vi "Actor Core.vi"(8 "error in":errorcluster, 11 "Create Test Channel View in":refnum<class "Edit Test Channel View.lvclass">) -> (0 "error out":errorcluster, 3 "Actor out":refnum<class "Actor.lvclass">)   [LabVIEW 2013, in "Edit Test Channel View.lvlib" / "Edit Test Channel View.lvclass"]
doc: "(<B>Filename</B>: Actor Framework.lvlib:Actor.lvclass:Actor Core.vi)\n\nReceives messages to the actor, reacts to them, and initiates any error handling that may shut the actor down.\n\nDescendant classes may override this VI to append parallel tasks for the actor to complete while it handles messages. Overrides use the Call Parent Method node."
uses:
  Edit Test Channel View.lvclass
  <vilib>/ActorFramework/Actor/Actor.lvclass
  <vilib>/ActorFramework/Actor/Actor.lvclass/Actor.ctl
  <vilib>/ActorFrameworkMVC/View Actor/View Actor.lvclass
  <vilib>/ActorFramework/Message Enqueuer/Message Enqueuer.lvclass/Message Enqueuer.ctl
  Edit Test Channel View.lvclass/Edit Test Channel View.ctl
  Models/Edit Test Channel Model Messages/Set Item Configurations Msg/Set Item Configurations Msg.lvclass/Set Item Configurations Msg.ctl
  <vilib>/Utility/miscctls.llb/LVPositionTypeDef.ctl
  <vilib>/ActorFrameworkMVC/UI Controller Messages/Move Subpanel Msg/Move Subpanel Msg.lvclass/Move Subpanel Msg.ctl
  <vilib>/ActorFrameworkMVC/UI Controller Messages/Insert Subpanel Msg/Insert Subpanel Msg.lvclass/Insert Subpanel Msg.ctl
  <vilib>/ActorFramework/Message Enqueuer/Init from Existing Queue.vi
  <vilib>/ActorFramework/Message Enqueuer/Enqueue.vi
  <vilib>/ActorFramework/Message Priority Queue/Priority Enqueue.vi
  <vilib>/ActorFramework/Message Enqueuer/Message Enqueuer.lvclass
  Models/Edit Test Channel Model Messages/Set Item Configurations Msg/Set Item Configurations Msg.lvclass
  Models/Edit Test Channel Model Messages/Load Test Channel Msg/Load Test Channel Msg.lvclass
  <vilib>/ActorFrameworkMVC/UI Controller Messages/Move Subpanel Msg/Move Subpanel Msg.lvclass
  <vilib>/ActorFrameworkMVC/UI Controller Messages/Insert Subpanel Msg/Insert Subpanel Msg.lvclass
  Models/Edit Test Channel Model Messages/Save Test Channel Msg/Save Test Channel Msg.lvclass
  Models/Test Channel Model Messages/Preview Test Channel Msg/Preview Test Channel Msg.lvclass
  Models/Test Channel Model Messages/Update Tiles Info Msg/Update Tiles Info Msg.lvclass
  Models/Test Channel Model Messages/Update Previous Button Visibility Msg/Update Previous Button Visibility Msg.lvclass
  Models/Test Channel Model Messages/Update Next Button Visibility Msg/Update Next Button Visibility Msg.lvclass
  Common/File IO/File IO.lvlib
  <vilib>/ActorFrameworkMVC/View Actor Messages/Get Model Enqueuer Msg/Get Model Enqueuer Msg.lvclass
  <vilib>/ActorFrameworkMVC/UI Controller Messages/Get Model Actor Enqueuer Msg/Get Model Actor Enqueuer Msg.lvclass
panel:
  in  "Cancel":bool
  in  "Save":bool
  out "Tab Control":enum32{"Basic Info"}(tab)
  in  "Channel Description":string caption="测试通道描述："
  in  "Channel Name":string caption="测试通道名称："
  in  "Channel ID":u16(ring) caption="测试通道ID：" items=["通道 1", "通道 2", "通道 3", "通道 4"]
  in  "Channel Sensor Name":u16(ring) caption="测试通道传感器：" items=["传感器 1", "传感器 2", "传感器 3", "传感器 4"]
  # "编辑测试通道"
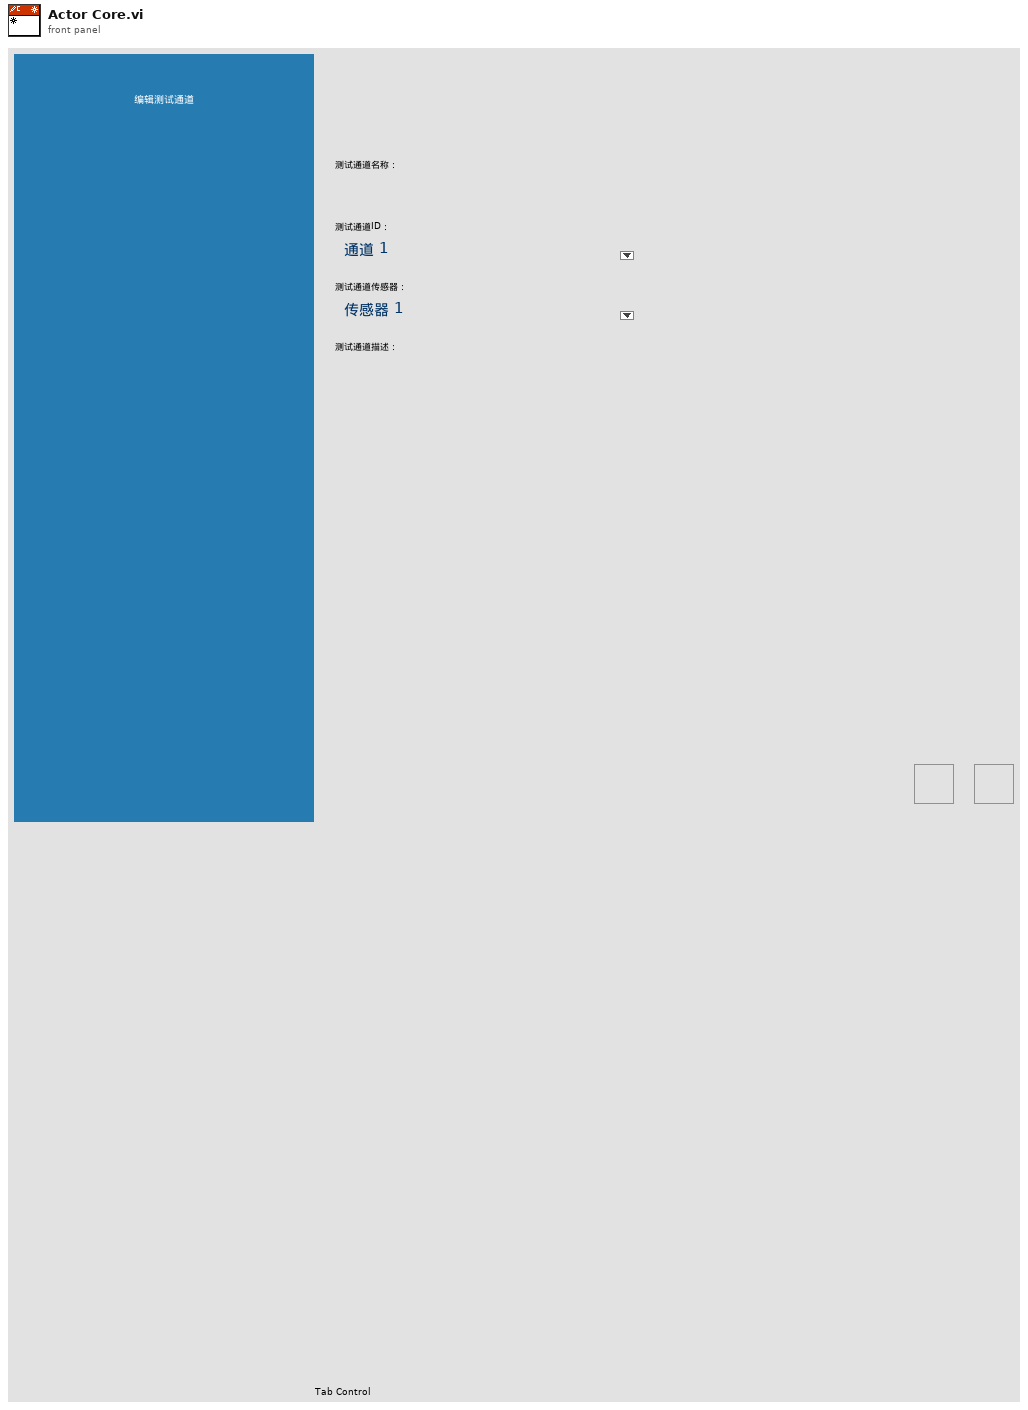
[diagram p1: front panel]
types:
  T1 = typedef "Edit Test Channel View.lvlib/Edit Test Channel View.lvclass/Events.ctl" = cluster{"Reinitialize All":refnum<user-event>}
  T2 = typedef "LVPositionTypeDef.ctl" = cluster{"Left":i32, "Top":i32}
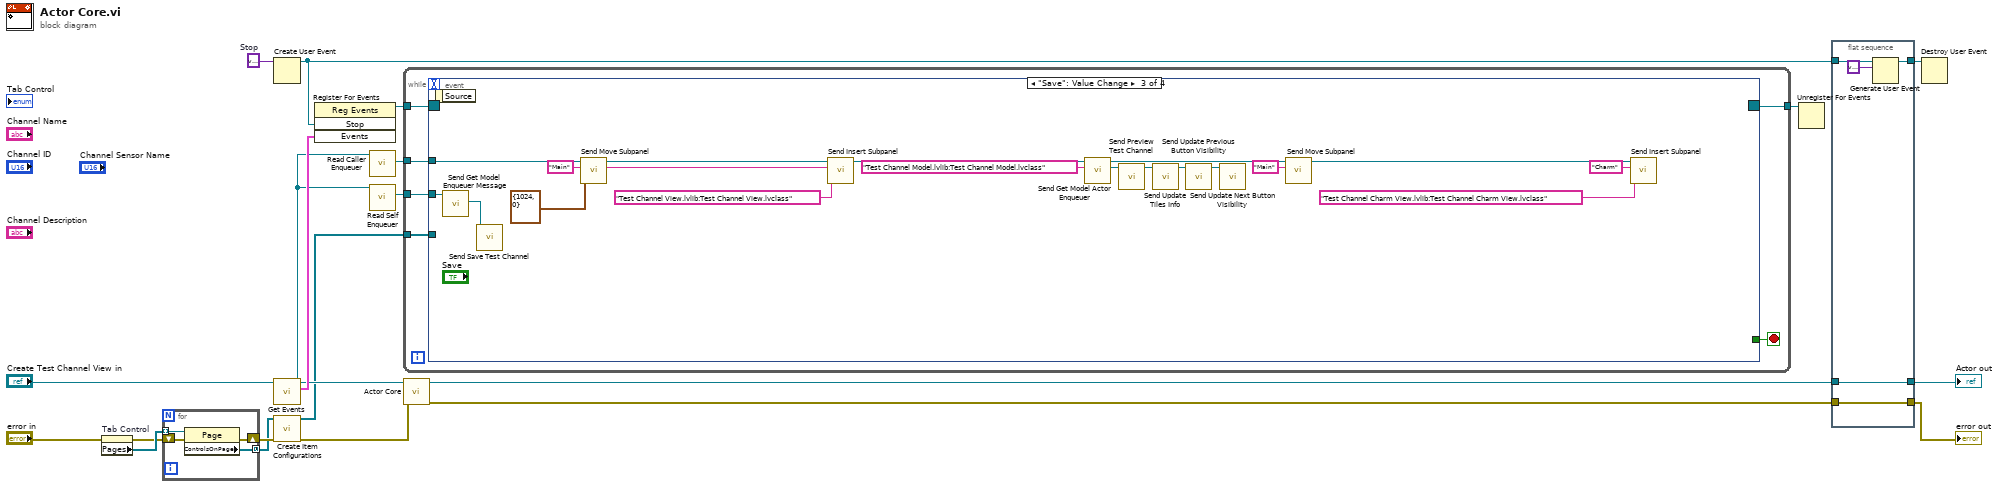
[diagram p0: block diagram]
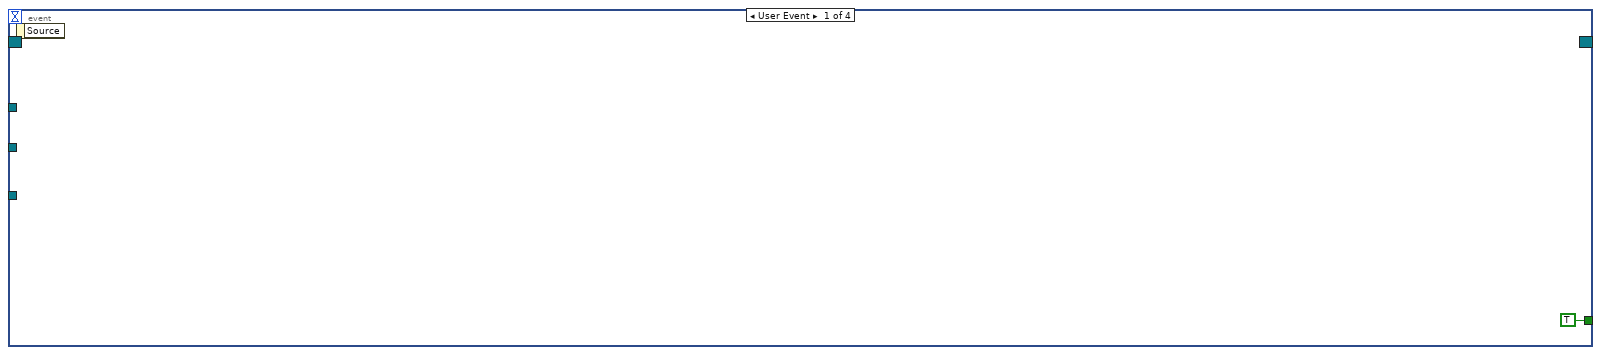
[diagram p2: hidden frame]
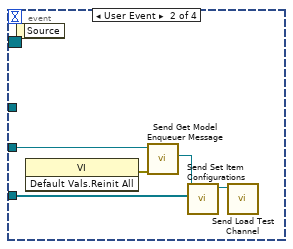
[diagram p3: hidden frame]
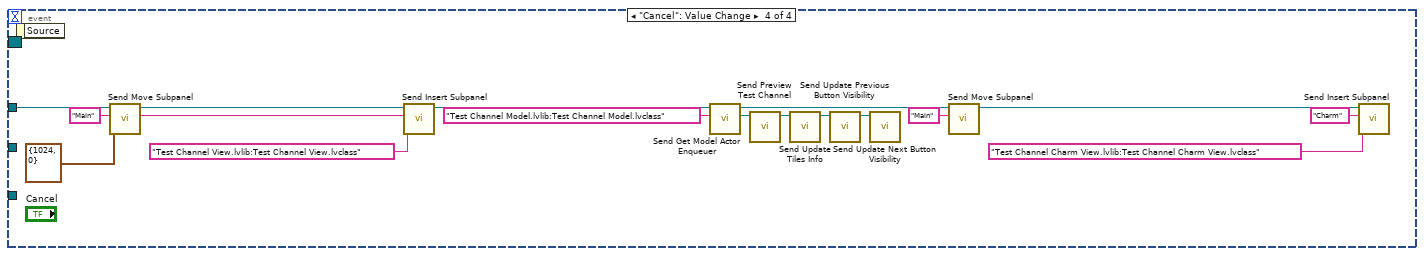
[diagram p4: hidden frame]
diagram:
  w21 = variant  # Stop
  n1 = property on="Tab Control" class="TabCtl (strict)"(error in="error in") -> (error out=w10:errorcluster, "Pages"=w11:refnum<vi>[])  [unwired: 1 in, 1 out]
  n2 = for {
    tunnel: w11 -> [w25] mode=indexing
    tunnel: [w24] -> w8 mode=concatenating
    shift-right: [w22] -> w9
    shift-left: w10 -> [w23]
    n3 = property class="Page"(reference=w25, error in=w23) -> (error out=w22:errorcluster, "ControlsOnPage"=w24:refnum<vi>[])  [unwired: 1 out]
  }
  n4 = Create User Event(user event datatype=w21) -> (user event=w14:refnum<user-event>)  [unwired: 1 in, 1 out]
  n5 = call "Get Events.vi"("Create Test Channel View in"="Create Test Channel View in") -> ("Events"=w13:T1, "Create Test Channel View out"=w4:refnum<class "Edit Test Channel View.lvclass">)  [unwired: 9 in]
  n6 = call "Create Item Configurations.vi"("error in (no error)"=w9, "Controls References"=w8) -> ("error out"=w3:errorcluster, "Item Configurations"=w1:refnum<class "Item Configuration.lvclass">[])  [unwired: 8 in]
  n7 = register-events(w14, w13) -> (reference out=w15:refnum<event-registration>)  [unwired: 2 in, 1 out]
  n8 = call <vilib>:"Read Caller Enqueuer.vi"("Actor"=w4) -> ("Caller Enqueuer"=w6:refnum<class "Message Enqueuer.lvclass">)  [unwired: 10 in]
  n9 = call <vilib>:"Read Self Enqueuer.vi"("Actor"=w4) -> ("Self Enqueuer"=w5:refnum<class "Message Enqueuer.lvclass">)  [unwired: 10 in]
  n10 = while {
    tunnel: [w31] -> w12
    tunnel: w15 -> [w29]
    tunnel: w6 -> [w28]
    tunnel: w5 -> [w27]
    tunnel: w1 -> [w26]
    stop <- w30 stop-if-true
    n11 = event shown="[2] \"Save\": Value Change" {
      selector: w29 -> [_ _ _ _]
      dyn-events: [_ _ _ _] -> w31
      timeout: _ -> [_ _ _ _]
      tunnel: [TRUE _ _ _] -> w30
      tunnel: w28 -> [_ _ w51 w68]
      tunnel: w27 -> [_ w34 w55 _]
      tunnel: w26 -> [_ w33 _ _]
      event User Event {
        n12 = event-data() -> ()  [unwired: 1 in, 1 out]
      }
      event User Event {
        n13 = event-data() -> ()  [unwired: 1 in, 1 out]
        n14 = invoke class="VI" method="Default Vals.Reinit All"() -> (error out=w37:errorcluster)  [unwired: 3 in, 2 out]
        n15 = call <vilib>:"Send Get Model Enqueuer Message.vi"("error in (no error)"=w37, "Message Enqueuer in"=w34) -> ("Reply"=w36:refnum<class "Message Enqueuer.lvclass">)  [unwired: 6 in, 3 out]
        n16 = call "Send Set Item Configurations.vi"("Item Configurations"=w33, "Message Enqueuer"=w36) -> ("Message Enqueuer out"=w35:refnum<class "Message Enqueuer.lvclass">)  [unwired: 8 in, 1 out]
        n17 = call "Send Load Test Channel.vi"("Message Enqueuer"=w35) -> ()  [unwired: 9 in, 2 out]
      }
      event "Save": Value Change {
        w41 = "Main" ("Subpanel Name")
        n18 = event-data() -> ()  [unwired: 1 in, 1 out]
        n19 = call <vilib>:"Send Get Model Enqueuer Message.vi"("Message Enqueuer in"=w55) -> ("Reply"=w38:refnum<class "Message Enqueuer.lvclass">)  [unwired: 7 in, 3 out]
        n20 = call "Send Save Test Channel.vi"("Message Enqueuer"=w38) -> ()  [unwired: 9 in, 2 out]
        n21 = call <vilib>:"Send Move Subpanel.vi"("Position (0,0)"=T2 {"Left"=1024, "Top"=0}, "Subpanel Name"=w41, "Message Enqueuer"=w51) -> ("Message Enqueuer out"=w43:refnum<class "Message Enqueuer.lvclass">)  [unwired: 7 in, 1 out]
        n22 = call <vilib>:"Send Insert Subpanel.vi"("View Name"="Test Channel View.lvlib:Test Channel View.lvclass" ("Subpanel Name"), "Subpanel Name"=w41, "Message Enqueuer"=w43) -> ("Message Enqueuer out"=w48:refnum<class "Message Enqueuer.lvclass">)  [unwired: 7 in, 1 out]
        n23 = call <vilib>:"Send Get Model Actor Enqueuer.vi"("Model Name"="Test Channel Model.lvlib:Test Channel Model.lvclass", "Message Enqueuer in"=w48) -> ("Reply"=w44:refnum<class "Message Enqueuer.lvclass">, "Message Enqueuer out"=w42:refnum<class "Message Enqueuer.lvclass">)  [unwired: 6 in, 2 out]
        n24 = call "Send Preview Test Channel.vi"("Message Enqueuer"=w44) -> ("Message Enqueuer out"=w47:refnum<class "Message Enqueuer.lvclass">)  [unwired: 9 in, 1 out]
        n25 = call "Send Update Tiles Info.vi"("Message Enqueuer"=w47) -> ("Message Enqueuer out"=w46:refnum<class "Message Enqueuer.lvclass">)  [unwired: 9 in, 1 out]
        n26 = call "Send Update Previous Button Visibility.vi"("Message Enqueuer"=w46) -> ("Message Enqueuer out"=w45:refnum<class "Message Enqueuer.lvclass">)  [unwired: 9 in, 1 out]
        n27 = call "Send Update Next Button Visibility.vi"("Message Enqueuer"=w45) -> ()  [unwired: 9 in, 2 out]
        n28 = call <vilib>:"Send Move Subpanel.vi"("Subpanel Name"="Main", "Message Enqueuer"=w42) -> ("Message Enqueuer out"=w52:refnum<class "Message Enqueuer.lvclass">)  [unwired: 8 in, 1 out]
        n29 = call <vilib>:"Send Insert Subpanel.vi"("View Name"="Test Channel Charm View.lvlib:Test Channel Charm View.lvclass", "Subpanel Name"="Charm", "Message Enqueuer"=w52) -> ()  [unwired: 7 in, 2 out]
      }
      event "Cancel": Value Change {
        w58 = "Main" ("Subpanel Name")
        n30 = event-data() -> ()  [unwired: 1 in, 1 out]
        n31 = call <vilib>:"Send Move Subpanel.vi"("Position (0,0)"=T2 {"Left"=1024, "Top"=0}, "Subpanel Name"=w58, "Message Enqueuer"=w68) -> ("Message Enqueuer out"=w60:refnum<class "Message Enqueuer.lvclass">)  [unwired: 7 in, 1 out]
        n32 = call <vilib>:"Send Insert Subpanel.vi"("View Name"="Test Channel View.lvlib:Test Channel View.lvclass" ("Subpanel Name"), "Subpanel Name"=w58, "Message Enqueuer"=w60) -> ("Message Enqueuer out"=w65:refnum<class "Message Enqueuer.lvclass">)  [unwired: 7 in, 1 out]
        n33 = call <vilib>:"Send Get Model Actor Enqueuer.vi"("Model Name"="Test Channel Model.lvlib:Test Channel Model.lvclass", "Message Enqueuer in"=w65) -> ("Reply"=w61:refnum<class "Message Enqueuer.lvclass">, "Message Enqueuer out"=w59:refnum<class "Message Enqueuer.lvclass">)  [unwired: 6 in, 2 out]
        n34 = call "Send Preview Test Channel.vi"("Message Enqueuer"=w61) -> ("Message Enqueuer out"=w64:refnum<class "Message Enqueuer.lvclass">)  [unwired: 9 in, 1 out]
        n35 = call "Send Update Tiles Info.vi"("Message Enqueuer"=w64) -> ("Message Enqueuer out"=w63:refnum<class "Message Enqueuer.lvclass">)  [unwired: 9 in, 1 out]
        n36 = call "Send Update Previous Button Visibility.vi"("Message Enqueuer"=w63) -> ("Message Enqueuer out"=w62:refnum<class "Message Enqueuer.lvclass">)  [unwired: 9 in, 1 out]
        n37 = call "Send Update Next Button Visibility.vi"("Message Enqueuer"=w62) -> ()  [unwired: 9 in, 2 out]
        n38 = call <vilib>:"Send Move Subpanel.vi"("Subpanel Name"="Main", "Message Enqueuer"=w59) -> ("Message Enqueuer out"=w69:refnum<class "Message Enqueuer.lvclass">)  [unwired: 8 in, 1 out]
        n39 = call <vilib>:"Send Insert Subpanel.vi"("View Name"="Test Channel Charm View.lvlib:Test Channel Charm View.lvclass", "Subpanel Name"="Charm", "Message Enqueuer"=w69) -> ()  [unwired: 7 in, 2 out]
      }
    }
  }
  n40 = call-parent "Actor Core.vi"("error in"=w3, "View Actor in"=w4) -> ("error out"=w18:errorcluster, "Actor out"=w19:refnum<class "Actor.lvclass">)  [unwired: 8 in]
  n41 = Unregister For Events(event registration refnum=w12) -> ()  [unwired: 1 in, 1 out]
  n42 = flat-sequence "Generate a stop event when the actor core stopped." {
    tunnel: w14 -> [w76]
    tunnel: [w74] -> w20
    tunnel: w19 -> [w73]
    tunnel: w18 -> [w72]
    tunnel: [w73] -> w17
    tunnel: [w72] -> w16
    frame #0 {
      n43 = Generate User Event(user event=w76, event data cluster=variant ("event data")) -> (user event out=w74:refnum<user-event>)  [unwired: 2 in, 1 out]
    }
  }
  n44 = Destroy User Event(user event=w20) -> ()  [unwired: 1 in, 1 out]
  "error out" <- w16
  "Actor out" <- w17
